vi "未命名 1 (子VI).vi"(1 "字符串":string) -> ()   [LabVIEW 2011]
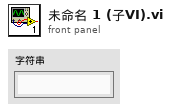
[diagram p1: front panel]
types:
  T1 = typedef "Sound Output Task ID.ctl" = u32
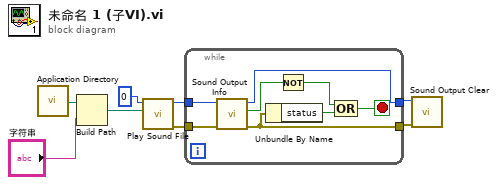
[diagram p0: block diagram]
diagram:
  n1 = call <vilib>:"Application Directory.vi"() -> ("Application Directory"=w3:path)
  n2 = Build Path(base path=w3, name or relative path="字符串") -> (appended path=w4:path)
  n3 = call <vilib>:"Play Sound File.vi"("path"=w4, "device ID"=u32 0) -> ("error out"=w6:errorcluster, "task ID"=w5:T1)  [unwired: 8 in]
  n4 = while {
    tunnel: w5 -> [w16]
    tunnel: w6 -> [w15]
    tunnel: [w10] -> w7
    tunnel: [w9] -> w8
    stop <- w11 stop-if-true
    n5 = call <vilib>:"Sound Output Info.vi"("error in (no error)"=w15, "task ID"=w16) -> ("error out"=w9:errorcluster, "is playing?"=w13:bool, "task ID out"=w10:T1)  [unwired: 6 in, 1 out]
    n6 = Unbundle By Name(w9) -> ("status"=w14:bool)
    n7 = Not(x=w13) -> (.not. x?=w12:bool)
    n8 = Compound Arithmetic op=OR(w12, w14) -> (w11:bool)
  }
  n9 = call <vilib>:"Sound Output Clear.vi"("error in (no error)"=w8, "task ID"=w7) -> ()  [unwired: 9 in, 1 out]
